vi "Kepco cfg current limit.vi"(8 "error in (no error)":errorcluster {"code" format="%.0x"}, 9 "Simulation":T1, 10 "Channel parsed command info":T2, 11 "input cluster":refnum<class "KepcoBOP.lvclass">) -> (0 "error out":errorcluster, 2 "new commands":string, 3 "output cluster":refnum<class "KepcoBOP.lvclass">)   [LabVIEW 2020, in "KepcoBOP.lvclass"]
uses:
  KepcoBOP.lvclass
  Shared/Device Driver/channel parsed cmd cluster.ctl
  shared/OnOffTypeDef.ctl
  KepcoBOP.lvclass/KepcoBOP.ctl
  shared/CompressAndUpdate(Poly)/CompressAndUpdate(Numeric).vi
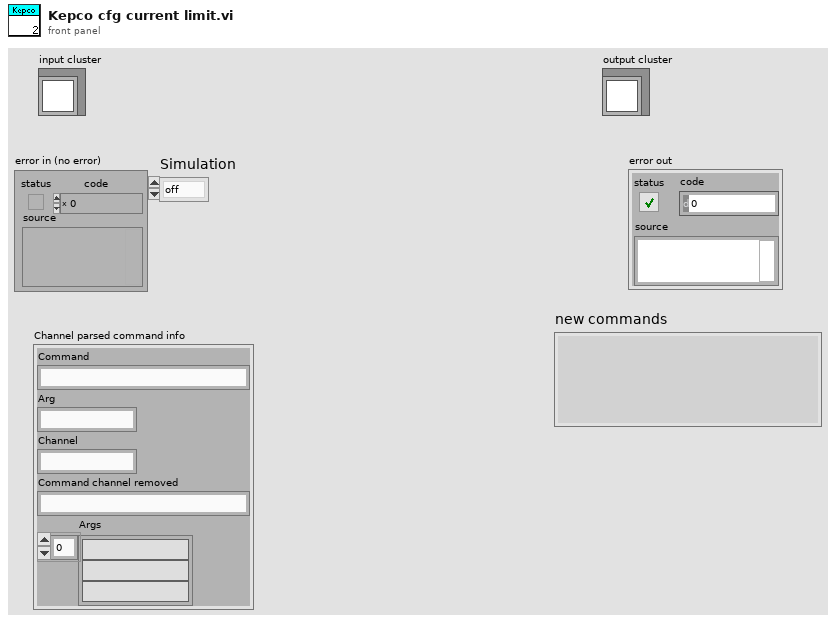
[diagram p1: front panel]
types:
  T1 = typedef "OnOffTypeDef.ctl" = enum16{"off", "on"}
  T2 = typedef "channel parsed cmd cluster.ctl" = cluster{"Command":string, "Arg":string, "Channel":string, "Command channel removed":string, "Args":string[]}
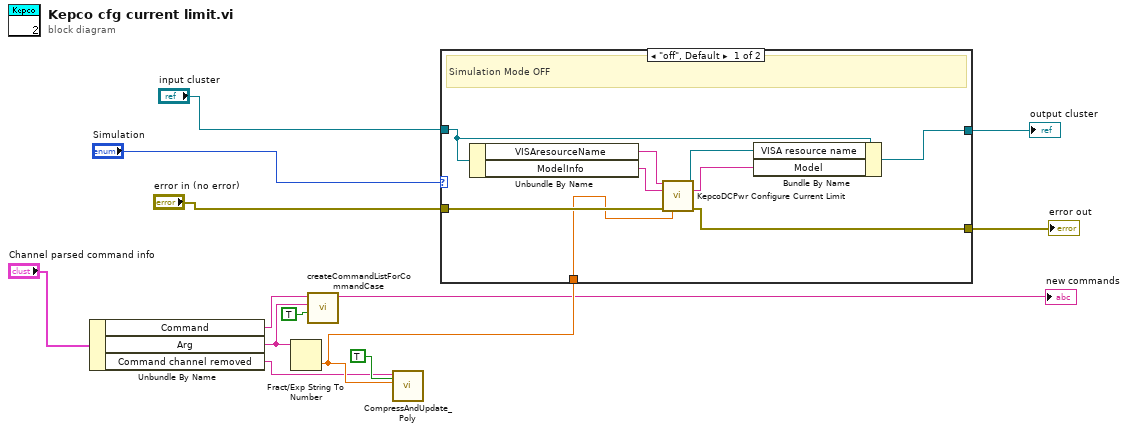
[diagram p0: block diagram]
diagram:
  n1 = Unbundle By Name("Channel parsed command info") -> ("Command"=w11:string, "Arg"=w13:string, "Command channel removed"=w1:string)
  n2 = Fract/Exp String To Number(string=w13) -> (number=w9:dbl)  [unwired: 3 in, 1 out]
  n3 = call "createCommandListForCommandCase.vi"("immediate Check (only once)"=TRUE, "setvalue"=w13, "command"=w11) -> ("new commands"=→"new commands":string)  [unwired: 8 in]
  n4 = call-poly "CompressAndUpdate_Poly.vi"("force CVT update (false)"=TRUE ("force CVT update"), "Numeric"=w9, "command or variable name"=w1) -> ()  [unwired: 8 in, 1 out]
  n5 = case shown="\"off\", Default" "Simulation" {
    tunnel: [w16 w23] -> w5
    tunnel: w9 -> [w17 _]
    tunnel: "input cluster" -> [w22 w24]
    tunnel: "error in (no error)" -> [w18 w23]
    tunnel: [w21 w24] -> w6
    frame "off", Default {
      # "Simulation Mode OFF"
      n6 = Unbundle By Name(w22) -> ("VISAresourceName"=w20:string, "ModelInfo"=w19:string)
      n7 = call "KepcoDCPwr Configure Current Limit.vi"("VISA Session"=w20, "Model In"=w19, "error in (no error)"=w18, "limit (0.0)"=w17) -> ("VISA Session Out"=w14:refnum<visa-resource-name>, "Model Out"=w15:string, "error out"=w16:errorcluster)  [unwired: 8 in, 1 out]
      n8 = Bundle By Name(cluster=w22, "VISA resource name"=w14, "Model"=w15) -> (w21:refnum<class "KepcoBOP.lvclass">)
    }
    frame "on" {
      # "Simulation Mode ON"
    }
  }
  "output cluster" <- w6
  "error out" <- w5
